vi "svx_Sound Write Waveform (DAQmx).vi"(0 "task ID":refnum<k21>, 1 "wave file path":path, 5 "waveform data":waveform(dbl)={"t0"=timestamp(0 s since 1904-01-01), "dt"=0.0, "Y"=[]}, 7 "bits per sample":i32=16, 11 "error in (no error)":errorcluster) -> (3 "dup wave file path":path, 4 "dup task ID":refnum<k21>, 6 "normalized data":waveform(dbl), 14 "SVT WAV info out":T1, 15 "error out":errorcluster)   [LabVIEW 2017]
uses:
  <vilib>/addons/_NISVFA/_Shared subVIs/Controls/SVT WAV Info.ctl
  <vilib>/addons/_NISVFA/_Shared subVIs/Controls/DAQ Coupling for SVT WAV Info.ctl
  <vilib>/addons/_NISVFA/_Shared subVIs/Controls/DAQ Polarity for SVT WAV Info.ctl
  <vilib>/addons/_NISVFA/_Shared subVIs/Controls/DAQ Terminal Configuration for SVT WAV Info.ctl
  <resource>/objmgr/daqmx.rc
panel:
  in  "SVT WAV info":T1
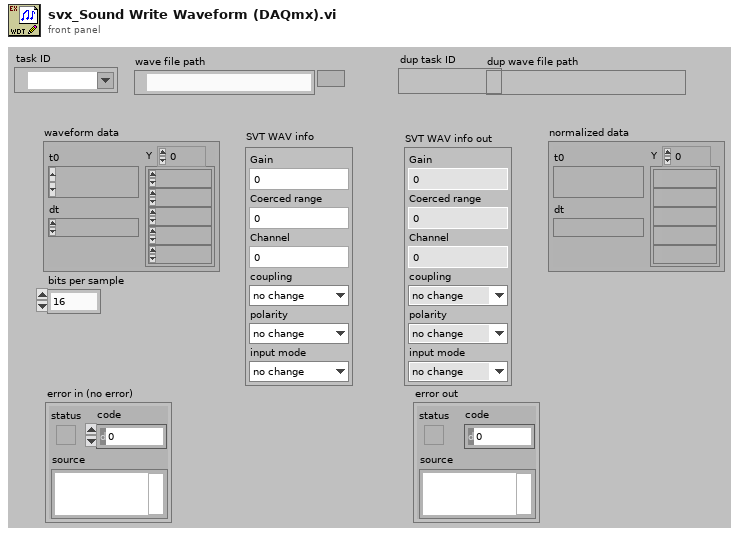
[diagram p1: front panel]
types:
  T1 = typedef "SVT WAV Info.ctl" = cluster{"Gain":u16, "Coerced range":u16, "Channel":u16, "coupling":T2, "polarity":T3, "input mode":T4}
  T2 = typedef "DAQ Coupling for SVT WAV Info.ctl" = enum16{"no change", "DC", "AC", "ground", "internal reference"}
  T3 = typedef "DAQ Polarity for SVT WAV Info.ctl" = enum16{"no change", "bipolar", "unipolar"}
  T4 = typedef "DAQ Terminal Configuration for SVT WAV Info.ctl" = enum16{"no change", "differential", "rse", "nrse", "pseudodifferential"}
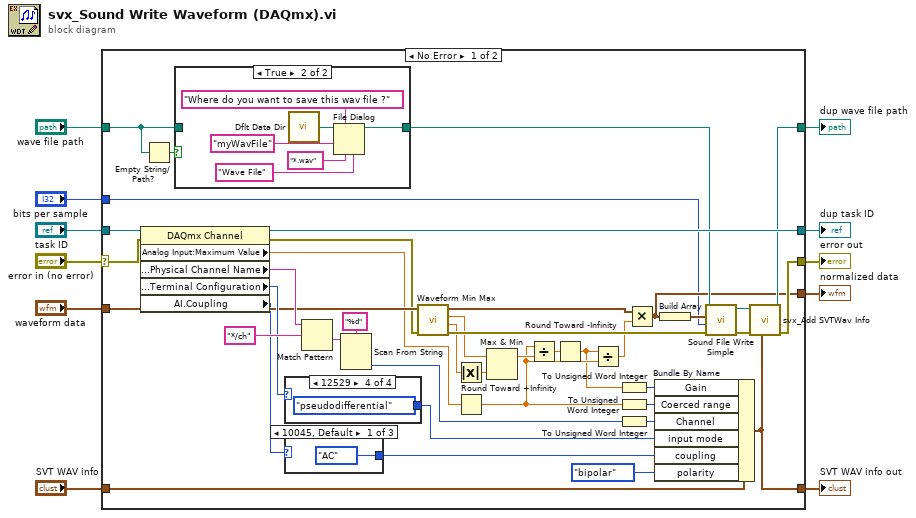
[diagram p0: block diagram]
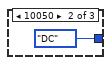
[diagram p2: hidden frame]
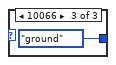
[diagram p3: hidden frame]
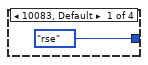
[diagram p4: hidden frame]
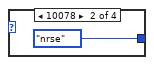
[diagram p5: hidden frame]
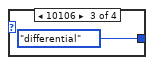
[diagram p6: hidden frame]
diagram:
  n1 = case shown="No Error" "error in (no error)" {
    selector: "error in (no error)" -> [w23 w70]
    tunnel: [w20 w68] -> w11
    tunnel: "SVT WAV info" -> [w52 w67]
    tunnel: [w51 w67] -> w9
    tunnel: "wave file path" -> [w49 w68]
    tunnel: "task ID" -> [w24 w69]
    tunnel: [w43 w69] -> w6
    tunnel: [w39 w70] -> w5
    tunnel: "waveform data" -> [w30 _]
    tunnel: [w14 _] -> w2
    tunnel: "bits per sample" -> [w13 _]
    frame No Error {
      n2 = property class="DAQmx Channel"(reference=w24, error in=w23) -> (reference out=w43:refnum<k21>, error out=w29:errorcluster, "Analog Input:Maximum Value"=w12:dbl, "General Properties:Physical Channel Name"=w48:tag, "Analog Input:General Properties:Input Configuration:Terminal Configuration"=w40:i32, "AI.Coupling"=w22:i32)
      n3 = Empty String/Path?(string/path=w49) -> (empty?=w50:bool)
      n4 = case shown="True" w50 {
        tunnel: w49 -> [w60 _]
        tunnel: [w60 w66] -> w21
        frame False {
        }
        frame True {
          n5 = call <vilib>:"Dflt Data Dir.vi"() -> ("App:Default Data Directory"=w64:path)
          n6 = File Dialog(4:"Wave File" ("pattern label"), 6:"*.wav" ("pattern"), 7:"Where do you want to save this wav file ?" ("prompt"), 9:"myWavFile" ("default name"), 11:w64) -> (3:w66:path)  [unwired: 2 in, 3 out]
        }
      }
      n7 = case shown="12529" w40 {
        tunnel: [DAQ_Terminal_Configuration_for_SVT_WAV_Info."rse" ("input mode") DAQ_Terminal_Configuration_for_SVT_WAV_Info."nrse" ("input mode") DAQ_Terminal_Configuration_for_SVT_WAV_Info."differential" ("input mode") DAQ_Terminal_Configuration_for_SVT_WAV_Info."pseudodifferential" ("input mode")] -> w19
        frame 10083, Default {
        }
        frame 10078 {
        }
        frame 10106 {
        }
        frame 12529 {
        }
      }
      n8 = case shown="10045, Default" w22 {
        tunnel: [DAQ_Coupling_for_SVT_WAV_Info."AC" ("coupling") DAQ_Coupling_for_SVT_WAV_Info."DC" ("coupling") DAQ_Coupling_for_SVT_WAV_Info."ground" ("coupling")] -> w38
        frame 10045, Default {
        }
        frame 10050 {
        }
        frame 10066 {
        }
      }
      n9 = Match Pattern(string=w48, regular expression="*/ch") -> (after substring=w45:string)  [unwired: 1 in, 3 out]
      n10 = Scan From String(format string="%d" ("Format String"), input string=w45) -> (output 1=w44:i32)  [unwired: 3 in, 3 out]
      n11 = call <vilib>:"Waveform Min Max.vi"("error in (no error)"=w29, "waveform in"=w30) -> ("error out"=w28:errorcluster, "Y min"=w26:dbl, "Y max"=w27:dbl, "waveform out"=w16:waveform(dbl))  [unwired: 4 in, 2 out]
      n12 = Absolute Value(x=w26) -> (abs(x)=w34:dbl)
      n13 = Round Toward +Infinity(x=w12) -> (ceil(x): smallest int >= x=w18:dbl)
      n14 = Max & Min(x=w27, y=w34) -> (max(x,y)=w32:dbl)  [unwired: 1 out]
      n15 = Divide(x=w18, y=w32) -> (x/y=w33:dbl)
      n16 = Round Toward -Infinity(1:w33) -> (0:w15:dbl)
      n17 = Divide(x=w15, y=w18) -> (x/y=w17:dbl)
      n18 = To Unsigned Word Integer(number=w15) -> (unsigned 16bit integer=w25:u16)
      n19 = To Unsigned Word Integer(number=w18) -> (unsigned 16bit integer=w31:u16)
      n20 = To Unsigned Word Integer(number=w44) -> (unsigned 16bit integer=w42:u16)
      n21 = Multiply(x=w16, y=w17) -> (x*y=w14:waveform(dbl))
      n22 = Bundle By Name(cluster=w52, "Gain"=w25, "Coerced range"=w31, "Channel"=w42, "input mode"=w19, "coupling"=w38, "polarity"=DAQ_Polarity_for_SVT_WAV_Info."bipolar") -> (w51:T1)
      n23 = Build Array(w14) -> (w35:waveform(dbl)[])
      n24 = call <vilib>:"Sound File Write Simple.vi"("error in (no error)"=w28, "bits per sample"=w13, "data"=w35, "path"=w21) -> ("error out"=w36:errorcluster, "path out"=w37:path)  [unwired: 6 in]
      n25 = call <vilib>:"svx_Add SVTWav Info.vi"("SVT WAV info"=w51, "error in (no error)"=w36, "wave file path in"=w37) -> ("error out"=w39:errorcluster, "wave file path"=w20:path)  [unwired: 7 in]
    }
    frame Error {
    }
  }
  "dup wave file path" <- w11
  "error out" <- w5
  "dup task ID" <- w6
  "SVT WAV info out" <- w9
  "normalized data" <- w2
